vi "Prompt on Selection Highlight.vi"(6 "String Reference In":refnum<vi>) -> (2 "Starting String":string)   [LabVIEW 2014]
doc: "This VI take a string reference and returns the highlighted selection."
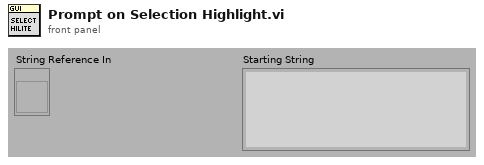
[diagram p1: front panel]
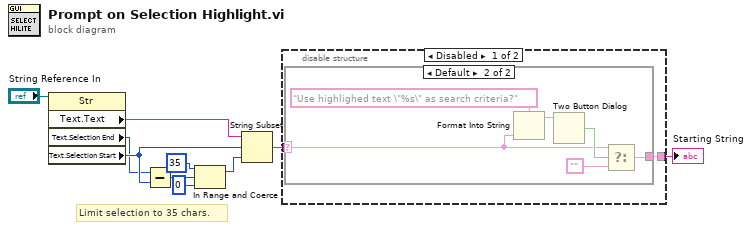
[diagram p0: block diagram]
diagram:
  # "Limit selection to 35 chars."
  n1 = property class="Str"(reference="String Reference In") -> ("Text.Text"=w4:string, "Text.Selection End"=w5:u32, "Text.Selection Start"=w6:u32)  [unwired: 1 in, 2 out]
  n2 = Subtract(x=w5, y=w6) -> (x-y=w8:u32)
  n3 = In Range and Coerce(upper limit=u32 35, x=w8, lower limit=u32 0) -> (coerced(x)=w9:u32)  [unwired: 1 out]
  n4 = String Subset(string=w4, offset (0)=w6, length (rest)=w9) -> (substring=w1:string)
  n5 = disable-structure shown="Disabled" {
    disable-tunnel: [w12 w19] -> w3
    disable-tunnel: w1 -> [w11 w19]
    frame Disabled {
      n6 = case shown="Default" w11 {
        selector: w11 -> [_ w13]
        tunnel: [_ w14] -> w12
        frame "" {
        }
        frame Default {
          n7 = Format Into String(format string="Use highlighed text \"%s\" as search criteria?", w13) -> (resulting string=w15:string)  [unwired: 2 in, 1 out]
          n8 = Two Button Dialog(message=w15) -> (T button?=w16:bool)  [unwired: 2 out]
          n9 = Select(t=w13, s=w16, f="") -> (s? t:f=w14:string)
        }
      }
    }
    frame Enabled {
    }
  }
  "Starting String" <- w3
